vi "CODMn通讯.vi"() -> ()   [LabVIEW 2016]
uses:
  <vilib>/Plasmionique/MB Master/MB Master.lvlib
  <vilib>/Utility/config.llb/NI_LVConfig.lvlib
panel:
  out "读取公式":u16[](array[numeric])
  out "读取参数":u16[](array[numeric])
  out "数据存储":u16[](array[numeric])
  out "温度":bool[](array[boolean])
  out "M输出点":bool[](array[boolean])
  out "ORP、时间":u16[](array[numeric])
  out "测量状态":u16[](array[numeric])
  out "通讯状态":bool
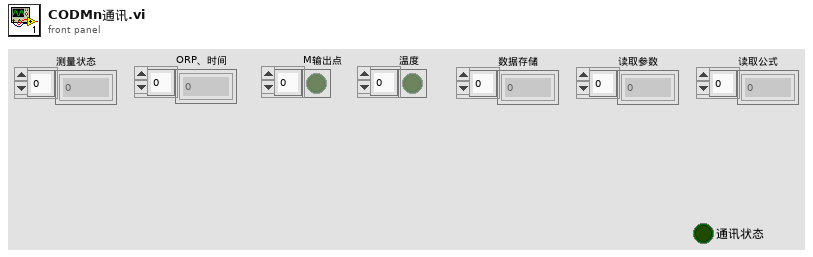
[diagram p1: front panel]
types:
  T1 = typedef "NI_LVConfig.lvlib/Config Data RefNum.ctl" = refnum<k1>
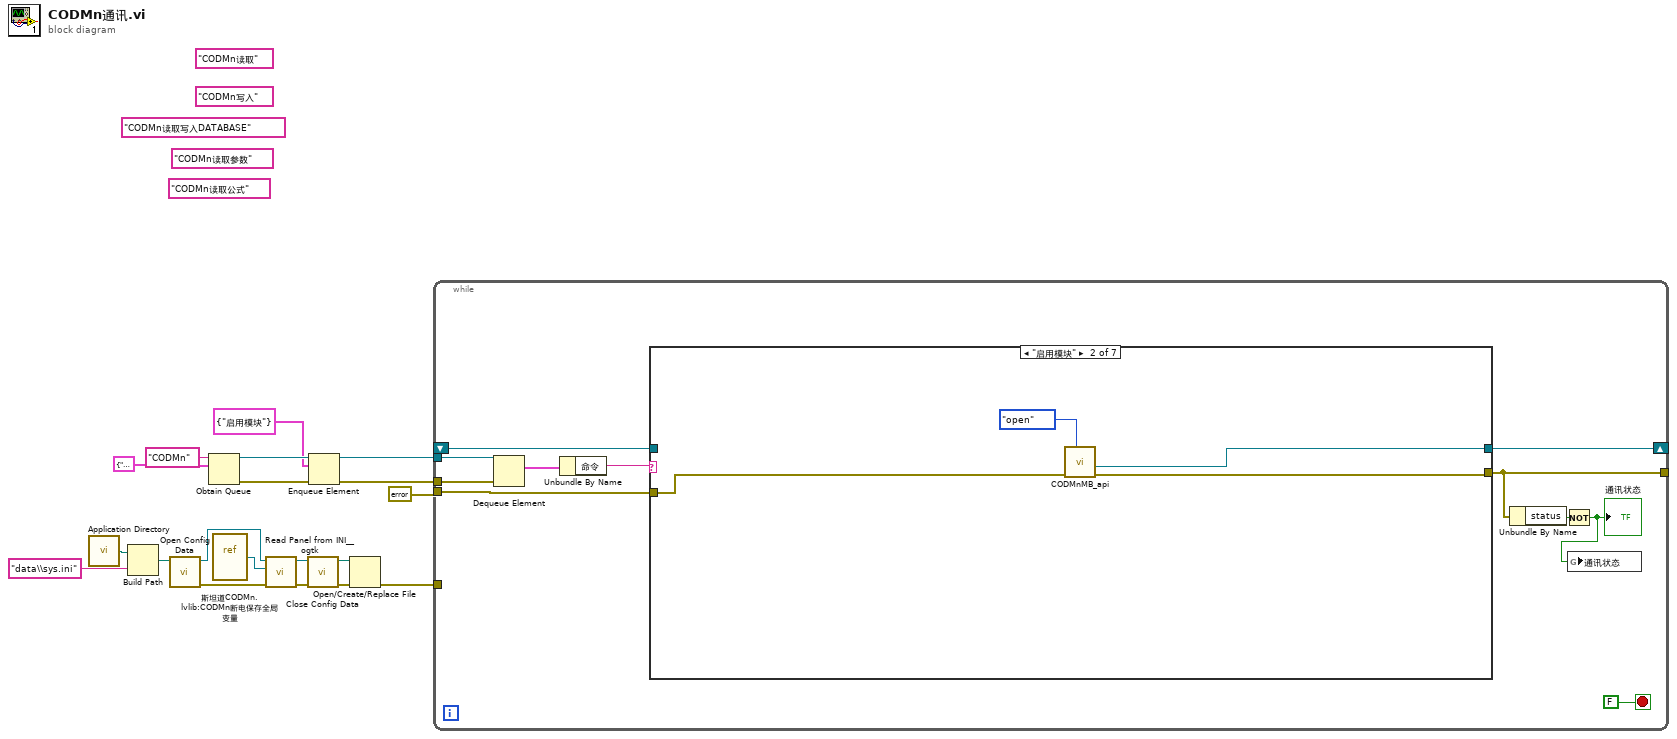
[diagram p0: block diagram]
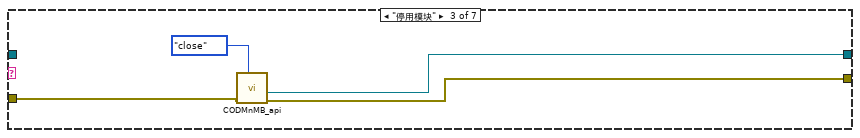
[diagram p3: hidden frame]
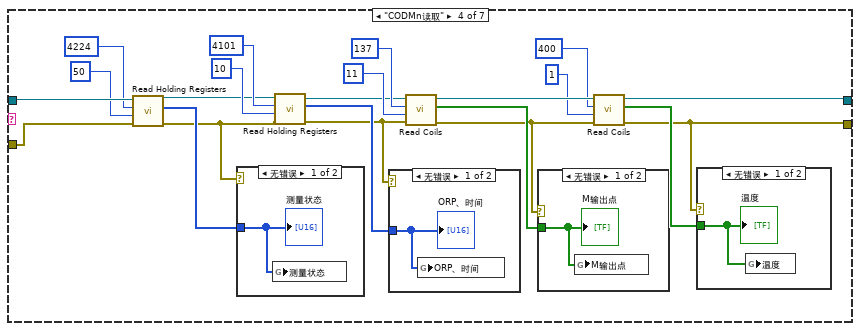
[diagram p4: hidden frame]
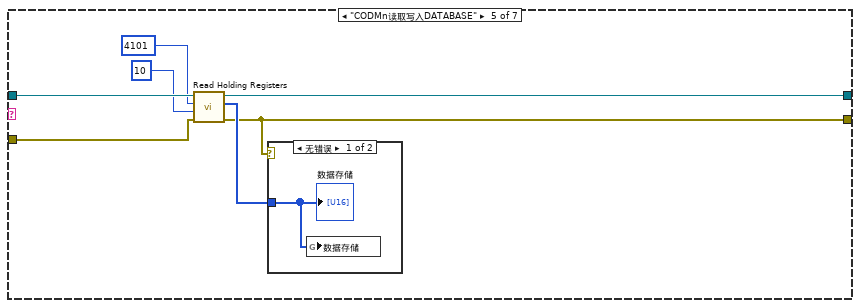
[diagram p9: hidden frame]
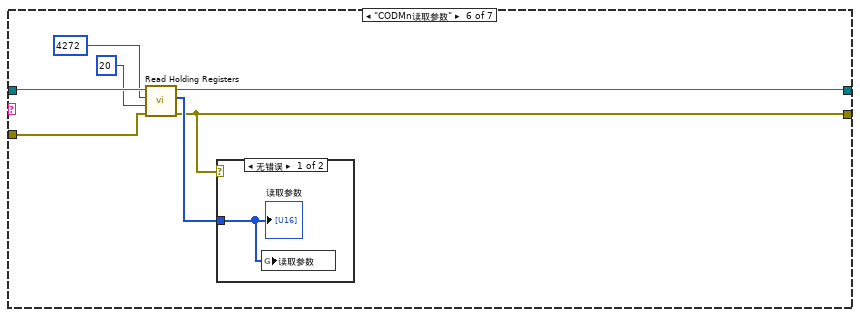
[diagram p11: hidden frame]
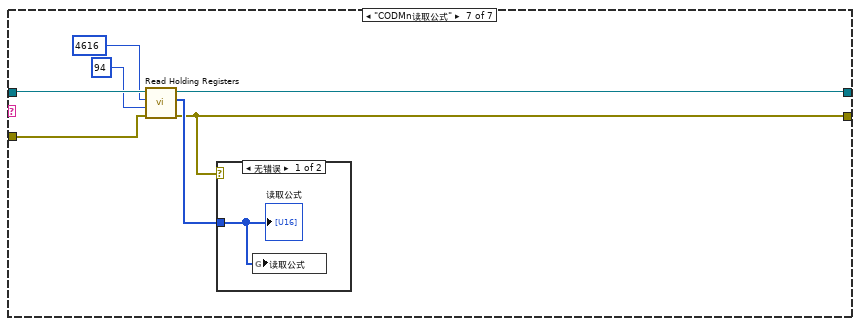
[diagram p13: hidden frame]
diagram:
  (unwired) "CODMn读取公式" ("名称（未命名）")
  (unwired) "CODMn读取写入DATABASE" ("名称（未命名）")
  (unwired) "CODMn读取参数" ("名称（未命名）")
  (unwired) "CODMn读取" ("名称（未命名）")
  (unwired) "CODMn写入" ("名称（未命名）")
  n1 = call <vilib>:"Application Directory.vi"() -> ("Application Directory"=w11:path)
  n2 = Build Path(base path=w11, name or relative path="data\\sys.ini" ("名称或相对路径")) -> (appended path=w9:path)
  n3 = call <vilib>:"Open Config Data.vi"("configuration file path"=w9) -> ("error out"=w5:errorcluster, "refnum"=w8:T1)  [unwired: 8 in, 1 out]
  n4 = Obtain Queue(name (unnamed)="CODMn" ("名称（未命名）"), element data type=cluster{"命令":string} {"命令"="启用模块"} ("元素")) -> (queue out=w16:refnum<queue>, error out=w15:errorcluster)  [unwired: 3 in, 1 out]
  n5 = vi-ref "斯坦道CODMn.lvlib:CODMn断电保存全局变量.vi"() -> (w7:refnum<vi>)
  n6 = call <userlib>:"Read Panel from INI__ogtk.vi"("error in (no error)"=w5, "VI ref"=w7, "refnum"=w8) -> ("error out"=w4:errorcluster, "refnum out"=w6:T1)  [unwired: 7 in]
  n7 = call <vilib>:"Close Config Data.vi"("error in (no error)"=w4, "refnum"=w6) -> ("error out"=w3:errorcluster, "file path"=w2:path)  [unwired: 8 in]
  n8 = Enqueue Element(queue=w16, element=cluster{"命令":string} {"命令"="启用模块"} ("元素"), error in (no error)=w15) -> (queue out=w14:refnum<queue>, error out=w13:errorcluster)  [unwired: 1 in, 1 out]
  n9 = Open/Create/Replace File(file path (use dialog)=w2, error in=w3) -> (error out=w1:errorcluster)  [unwired: 4 in, 2 out]
  n10 = while {
    tunnel: w14 -> [w29]
    tunnel: w13 -> [w28]
    tunnel: [w20] -> _
    shift-right: [w24] -> _
    shift-left: _ -> [w23]
    tunnel: errorcluster {"status"=FALSE, "code"=0, "source"=""} ("error out") -> [w22]
    tunnel: w1 -> [_]
    stop <- FALSE stop-if-true
    n11 = Dequeue Element(queue=w29, error in (no error)=w28) -> (element=w27:cluster{"命令":string})  [unwired: 1 in, 3 out]
    n12 = Unbundle By Name(w27) -> ("命令"=w26:string)
    n13 = case shown="\"启用模块\"" w26 {
      tunnel: [w32 w33 w37 w48 w69 w76 w86] -> w24
      tunnel: [w31 w36 w38 w41 w67 w75 w85] -> w20
      tunnel: w23 -> [w32 _ _ w62 w73 w81 w89]
      tunnel: w22 -> [w31 w34 w39 w61 w70 w80 w88]
      frame Default {
      }
      frame "启用模块" {
        n14 = call "CODMnMB_api.vi"("STEP"=enum16{"open", "read", "write", "close"}."open", "Error in"=w34) -> ("error out"=w36:errorcluster, "MB session out"=w33:refnum<class "MB_Master.lvclass">)  [unwired: 6 in, 2 out]
      }
      frame "停用模块" {
        n15 = call "CODMnMB_api.vi"("STEP"=enum16{"open", "read", "write", "close"}."close", "Error in"=w39) -> ("error out"=w38:errorcluster, "MB session out"=w37:refnum<class "MB_Master.lvclass">)  [unwired: 6 in, 2 out]
      }
      frame "CODMn读取" {
        n16 = call <vilib>:"Read Holding Registers.vi"("error in (no error)"=w61, "quantity"=u16 50 ("number of holding registers"), "starting address"=u16 4224, "MB session in"=w62) -> ("error out"=w52:errorcluster, "Registers"=w58:u16[], "MB session out"=w53:refnum<class "MB_Master.lvclass">)  [unwired: 5 in]
        n17 = case shown="无错误" w52 {
          tunnel: w58 -> [w66 _]
          frame No Error {
            n18 = global write "COD读取DATA全局.vi" "测量状态"(w66) -> ()
            "测量状态" <- w66
          }
          frame Error {
          }
        }
        n19 = call <vilib>:"Read Holding Registers.vi"("error in (no error)"=w52, "quantity"=u16 10, "starting address"=u16 4101, "MB session in"=w53) -> ("error out"=w47:errorcluster, "Registers"=w51:u16[], "MB session out"=w50:refnum<class "MB_Master.lvclass">)  [unwired: 5 in]
        n20 = case shown="无错误" w47 {
          tunnel: w51 -> [w65 _]
          frame No Error {
            n21 = global write "COD读取DATA全局.vi" "ORP、时间"(w65) -> ()
            "ORP、时间" <- w65
          }
          frame Error {
          }
        }
        n22 = call <vilib>:"Read Coils.vi"("error in (no error)"=w47, "quantity"=u16 11, "starting address"=u16 137, "MB session in"=w50) -> ("error out"=w45:errorcluster, "Coils"=w46:bool[], "MB session out"=w49:refnum<class "MB_Master.lvclass">)  [unwired: 5 in]
        n23 = case shown="无错误" w45 {
          tunnel: w46 -> [w64 _]
          frame No Error {
            n24 = global write "COD读取DATA全局.vi" "M输出点"(w64) -> ()
            "M输出点" <- w64
          }
          frame Error {
          }
        }
        n25 = call <vilib>:"Read Coils.vi"("error in (no error)"=w45, "quantity"=u16 1, "starting address"=u16 400, "MB session in"=w49) -> ("error out"=w41:errorcluster, "Coils"=w42:bool[], "MB session out"=w48:refnum<class "MB_Master.lvclass">)  [unwired: 5 in]
        n26 = case shown="无错误" w41 {
          tunnel: w42 -> [w63 _]
          frame No Error {
            n27 = global write "COD读取DATA全局.vi" "温度"(w63) -> ()
            "温度" <- w63
          }
          frame Error {
          }
        }
      }
      frame "CODMn读取写入DATABASE" {
        n28 = call <vilib>:"Read Holding Registers.vi"("error in (no error)"=w70, "quantity"=u16 10 ("number of holding registers"), "starting address"=u16 4101, "MB session in"=w73) -> ("error out"=w67:errorcluster, "Registers"=w68:u16[], "MB session out"=w69:refnum<class "MB_Master.lvclass">)  [unwired: 5 in]
        n29 = case shown="无错误" w67 {
          tunnel: w68 -> [w74 _]
          frame No Error {
            n30 = global write "COD读取DATA全局.vi" "数据存储"(w74) -> ()
            "数据存储" <- w74
          }
          frame Error {
          }
        }
      }
      frame "CODMn读取参数" {
        n31 = call <vilib>:"Read Holding Registers.vi"("error in (no error)"=w80, "quantity"=u16 20 ("number of holding registers"), "starting address"=u16 4272, "MB session in"=w81) -> ("error out"=w75:errorcluster, "Registers"=w77:u16[], "MB session out"=w76:refnum<class "MB_Master.lvclass">)  [unwired: 5 in]
        n32 = case shown="无错误" w75 {
          tunnel: w77 -> [w82 _]
          frame No Error {
            n33 = global write "COD读取DATA全局.vi" "读取参数"(w82) -> ()
            "读取参数" <- w82
          }
          frame Error {
          }
        }
      }
      frame "CODMn读取公式" {
        n34 = call <vilib>:"Read Holding Registers.vi"("error in (no error)"=w88, "quantity"=u16 94 ("number of holding registers"), "starting address"=u16 4616, "MB session in"=w89) -> ("error out"=w85:errorcluster, "Registers"=w87:u16[], "MB session out"=w86:refnum<class "MB_Master.lvclass">)  [unwired: 5 in]
        n35 = case shown="无错误" w85 {
          tunnel: w87 -> [w90 _]
          frame No Error {
            n36 = global write "COD读取DATA全局.vi" "读取公式"(w90) -> ()
            "读取公式" <- w90
          }
          frame Error {
          }
        }
      }
    }
    n37 = Unbundle By Name(w20) -> ("status"=w25:bool)
    n38 = Not(x=w25) -> (.not. x?=w21:bool)
    "通讯状态" <- w21
    n39 = global write "COD读取DATA全局.vi" "通讯状态"(w21) -> ()
  }
